vi "PL_Spectrum_detailed1.vi"() -> ()   [LabVIEW 2012]
uses:
  <vilib>/Utility/file.llb/Write To Spreadsheet File (DBL).vi
  <vilib>/Instr/_visa.llb/VISA Configure Serial Port (Instr).vi
  <vilib>/Analysis/baseanly.llb/Mean (DBL).vi
  <vilib>/Analysis/NI_AALBase.lvlib
panel:
  out "Current Wavelength (nm)":string
  out "Grating":string
  out "Scan Speed (nm/min)":string
  in  "Scan Speed (nm/min)":dbl
  in  "Scan Grating":dbl
  out "XY Graph":cluster{"Y":dbl[], "Y":dbl[]}[](graph)
  in  "End Wavelength (nm)":dbl
  in  "Start Wavelength (nm)":dbl
  in  "Resolution (nm)":dbl
  in  "Detector Input":T1
  in  "stop (T)":bool=TRUE
  in  "Resource name":refnum<visa-resource-name>
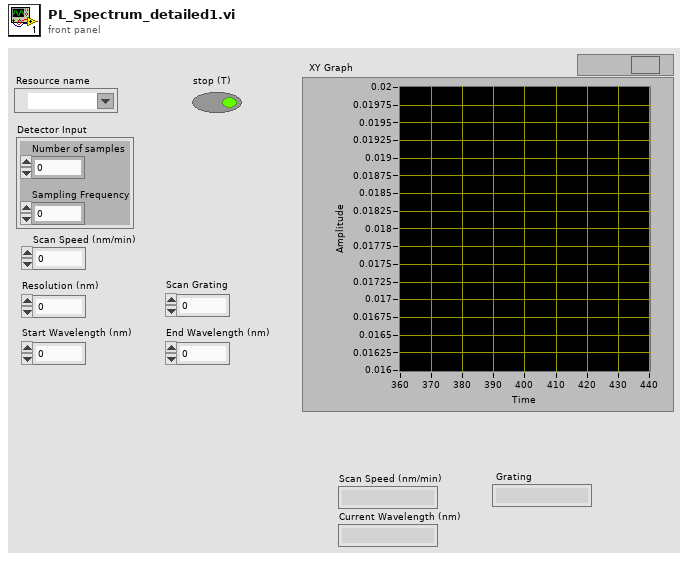
[diagram p1: front panel]
types:
  T1 = cluster{"Number of samples":i32, "Sampling Frequency":dbl}
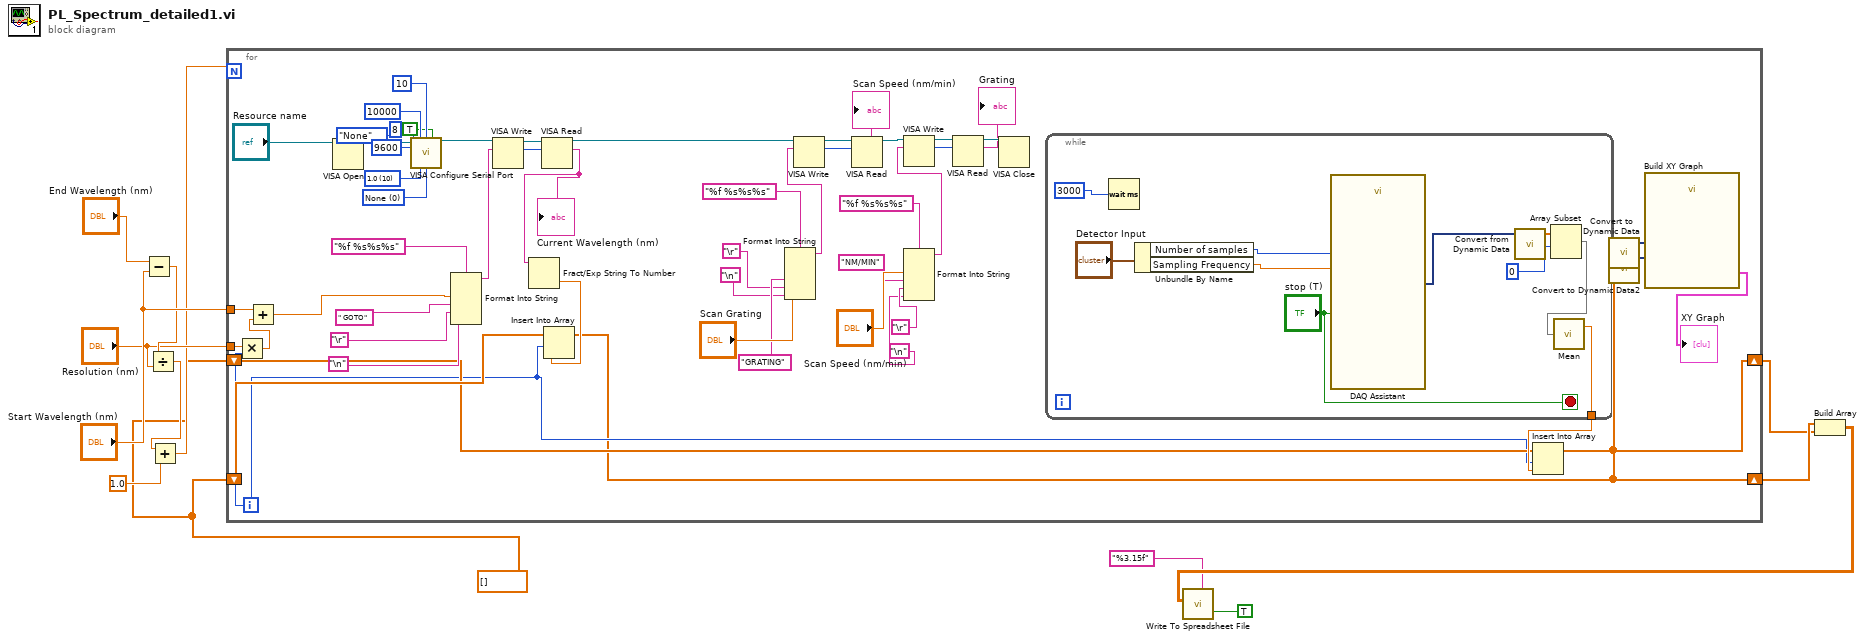
[diagram p0: block diagram]
diagram:
  w5 = dbl[] [] ("array")
  n1 = Subtract(x="End Wavelength (nm)", y="Start Wavelength (nm)") -> (x-y=w10:dbl)
  n2 = Divide(x=w10, y="Resolution (nm)") -> (x/y=w8:dbl)
  n3 = Add(x=w8, y=1.0) -> (x+y=w6:dbl)
  n4 = for {
    N: w6 -> [_]
    shift-right: [w40] -> w4
    shift-left: w5 -> [w48]
    tunnel: "Resolution (nm)" -> [w47]
    tunnel: "Start Wavelength (nm)" -> [w46]
    shift-right: [w38] -> w3
    shift-left: w5 -> [w43]
    i -> [w42]
    w56 = u16 0 items=["None", "XON/XOFF", "RTS/CTS", "XON/XOFF & RTS/CTS", "DTR/DSR", "XON/XOFF & DTR/DSR"] ("flow control (0:none)")
    w57 = u16 10 items=["1.0"=10, "1.5"=15, "2.0"=20] ("stop bits (10: 1 bit)")
    n5 = Multiply(x=w47, y=w42) -> (x*y=w49:dbl)
    n6 = Add(x=w46, y=w49) -> (x+y=w36:dbl)
    n7 = VISA Open(VISA resource name="Resource name") -> (VISA resource name=w61:refnum<visa-resource-name>)  [unwired: 4 in, 1 out]
    n8 = call-poly "VISA Configure Serial Port"("VISA resource name"=w61, "timeout (10sec)"=u32 10000, "termination char\n(0xA = '\\n' = LF)"=u8 10 ("termination char\n(0xA = '\\n' = LF)"), "Enable Termination\nChar (T)"=TRUE ("Enable Termination\nChar (T)"), "baud rate (9600)"=u32 9600, "data bits (8)"=u16 8, "parity (0:none)"=enum16{"None", "Odd", "Even", "Mark", "Space"}."None", "stop bits (10: 1 bit)"=w57, "flow control (0:none)"=w56) -> ("VISA resource name out"=w51:refnum<visa-resource-name>)  [unwired: 5 in, 1 out]
    n9 = Format Into String(format string="%f %s%s%s", w36, " GOTO" ("String"), "\r", "\n") -> (resulting string=w52:string)  [unwired: 2 in, 1 out]
    n10 = VISA Write(VISA resource name=w51, write buffer=w52) -> (VISA resource name out=w63:refnum<visa-resource-name>, return count=w62:u32)  [unwired: 1 in, 1 out]
    n11 = VISA Read(VISA resource name=w63, byte count=w62) -> (VISA resource name out=w14:refnum<visa-resource-name>, read buffer=w19:string)  [unwired: 1 in, 2 out]
    "Current Wavelength (nm)" <- w19
    n12 = Fract/Exp String To Number(string=w19) -> (number=w45:dbl)  [unwired: 3 in, 1 out]
    n13 = Insert Into Array(array=w48, index=w42, new element=w45) -> (w40:dbl[])
    n14 = Format Into String(format string="%f %s%s%s", "Scan Grating", "GRATING" ("input 2"), "\r", "\n") -> (resulting string=w34:string)  [unwired: 2 in, 1 out]
    n15 = VISA Write(VISA resource name=w14, write buffer=w34) -> (VISA resource name out=w35:refnum<visa-resource-name>, return count=w25:u32)  [unwired: 1 in, 1 out]
    n16 = VISA Read(VISA resource name=w35, byte count=w25) -> (VISA resource name out=w30:refnum<visa-resource-name>, read buffer=→"Scan Speed (nm/min)":string)  [unwired: 1 in, 2 out]
    n17 = Format Into String(format string="%f %s%s%s", "Scan Speed (nm/min)", "NM/MIN" ("input 2"), "\r", "\n") -> (resulting string=w26:string)  [unwired: 2 in, 1 out]
    n18 = VISA Write(VISA resource name=w30, write buffer=w26) -> (VISA resource name out=w29:refnum<visa-resource-name>, return count=w24:u32)  [unwired: 1 in, 1 out]
    n19 = VISA Read(VISA resource name=w29, byte count=w24) -> (VISA resource name out=w28:refnum<visa-resource-name>, read buffer=→"Grating":string)  [unwired: 1 in, 2 out]
    n20 = VISA Close(VISA resource name=w28) -> ()  [unwired: 1 in, 1 out]
    n21 = while {
      tunnel: [w73] -> w44
      stop <- "stop (T)" stop-if-true
      n22 = Wait (ms)(milliseconds to wait=u32 3000) -> ()  [unwired: 1 out]
      n23 = Unbundle By Name("Detector Input") -> ("Number of samples"=w70:i32, "Sampling Frequency"=w69:dbl)
      n24 = call "DAQ Assistant"("rate"=w69, "number of samples"=w70, "stop (T)"="stop (T)") -> ("data"=w77:dynamicdata)  [unwired: 14 in, 2 out]
      n25 = call "Convert from Dynamic Data"("Dynamic Data Type"=w77) -> ("Array"=w76:dbl[])  [unwired: 3 in]
      n26 = Array Subset(array=w76, index=0) -> (w75:dbl[])  [unwired: 1 in]
      n27 = call-poly <vilib>:"Mean.vi"("X"=w75) -> ("mean"=w73:dbl)  [unwired: 1 out]
    }
    n28 = Insert Into Array(array=w43, index=w42, new element=w44) -> (w38:dbl[])
    n29 = call "Convert to Dynamic Data"("Array"=w40) -> ("Dynamic Data Type"=w39:dynamicdata)  [unwired: 3 in]
    n30 = call "Convert to Dynamic Data2"("Array"=w38) -> ("Dynamic Data Type"=w37:dynamicdata)  [unwired: 3 in]
    n31 = call "Build XY Graph"("Y Input"=w37, "X Input"=w39) -> ("XY Graph"=→"XY Graph":cluster{"Y":dbl[], "Y":dbl[]}[])  [unwired: 8 in, 1 out]
  }
  n32 = Build Array(w4, w3) -> (w2:dbl[][])
  n33 = call-poly <vilib>:"Write To Spreadsheet File.vi"("transpose? (no:F)"=TRUE, "format (%.3f)"="%3.15f" ("format string"), "2D data"=w2) -> ()  [unwired: 5 in, 1 out]
